vi "ReadSlotNode.vi"(8 "Error In":errorcluster, 11 "Slot Node In":refnum<k20>) -> (0 "Error Out":errorcluster, 2 "Slot Configuration":T1, 3 "Slot Node Out":refnum<k20>)   [LabVIEW 2012]
uses:
  SlotConfiguration.ctl
  BankConfiguration.ctl
  <vilib>/xml/NI_XML.lvlib
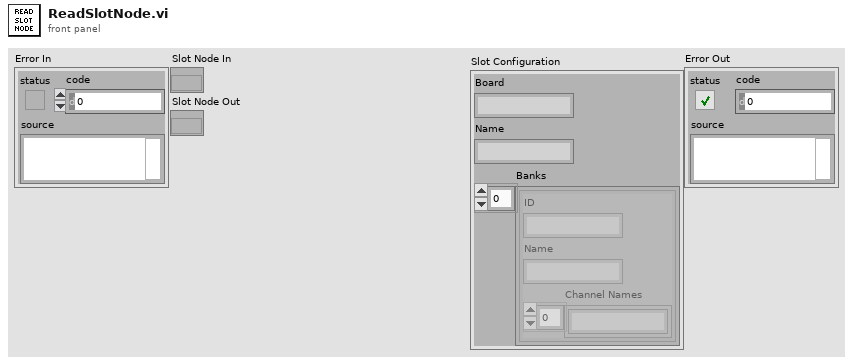
[diagram p1: front panel]
types:
  T1 = typedef "SlotConfiguration.ctl" = cluster{"Board":string, "Name":string, "Banks":T2[]}
  T2 = typedef "BankConfiguration.ctl" = cluster{"ID":string, "Name":string, "Channel Names":string[]}
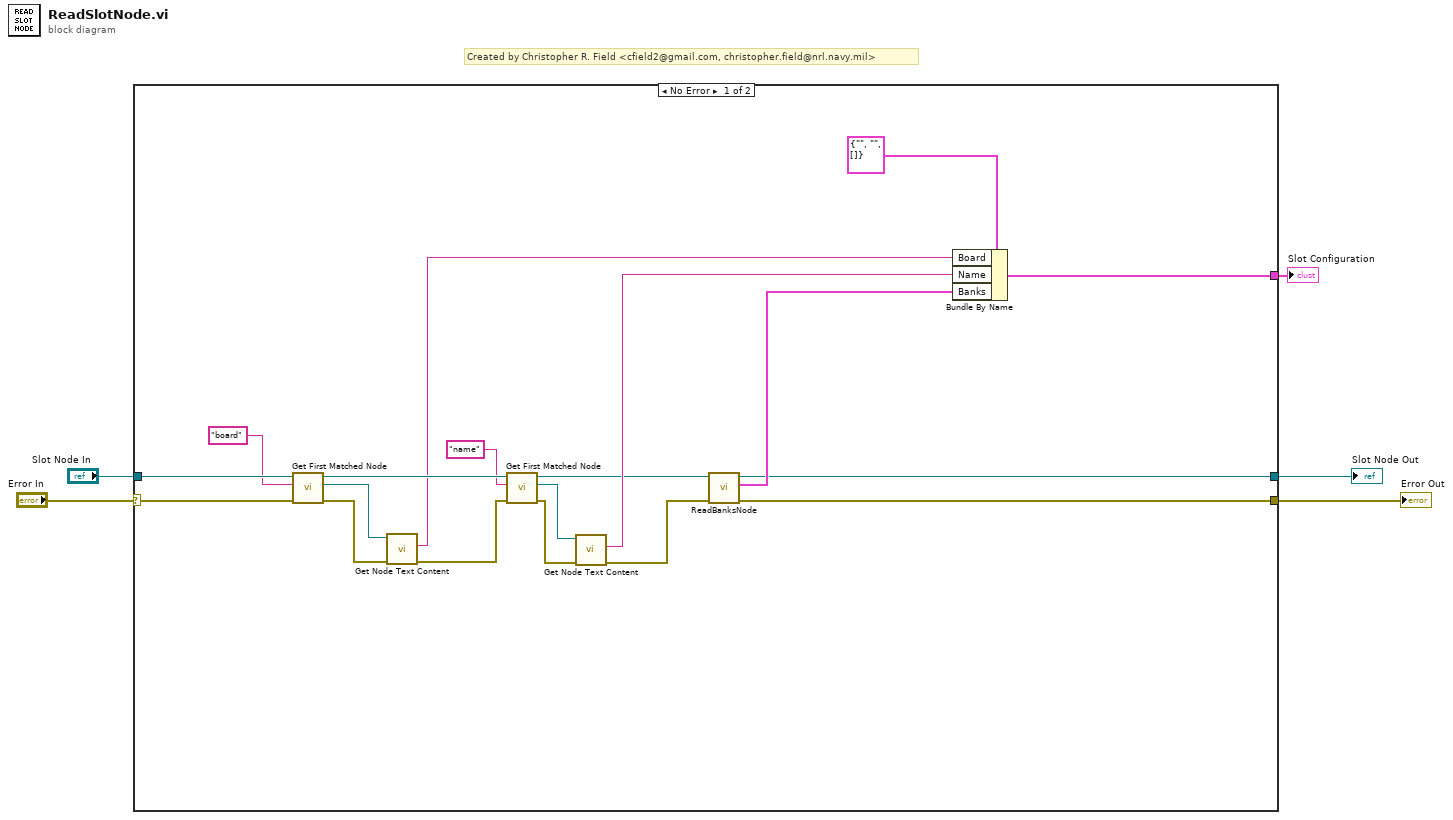
[diagram p0: block diagram]
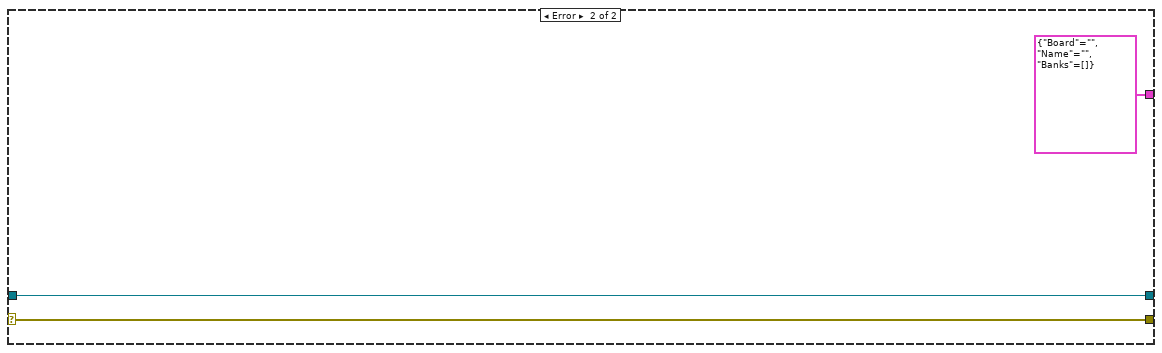
[diagram p2: hidden frame]
diagram:
  # "Created by Christopher R. Field <cfield2@gmail.com, christopher.field@nrl.navy.mil>"
  n1 = case shown="No Error" "Error In" {
    selector: "Error In" -> [w23 w26]
    tunnel: "Slot Node In" -> [w24 w27]
    tunnel: [w8 T1 {"Board"="", "Name"="", "Banks"=[]} ("Slot Configuration")] -> w3
    tunnel: [w7 w27] -> w1
    tunnel: [w6 w26] -> w2
    frame No Error {
      n2 = call <vilib>:"Get First Matched Node.vi"("error in (no error)"=w23, "XPath expression"="board", "node in"=w24) -> ("error out"=w20:errorcluster, "node result"=w21:refnum<k20>, "node out"=w19:refnum<k20>)  [unwired: 6 in]
      n3 = call <vilib>:"Get Node Text Content.vi"("error in (no error)"=w20, "node in"=w21) -> ("error out"=w17:errorcluster, "node text"=w13:string)  [unwired: 7 in, 1 out]
      n4 = call <vilib>:"Get First Matched Node.vi"("error in (no error)"=w17, "XPath expression"="name", "node in"=w19) -> ("error out"=w16:errorcluster, "node result"=w15:refnum<k20>, "node out"=w11:refnum<k20>)  [unwired: 6 in]
      n5 = call <vilib>:"Get Node Text Content.vi"("error in (no error)"=w16, "node in"=w15) -> ("error out"=w10:errorcluster, "node text"=w12:string)  [unwired: 7 in, 1 out]
      n6 = call "ReadBanksNode.vi"("Error In"=w10, "Slot Node In"=w11) -> ("Error Out"=w6:errorcluster, "Banks"=w9:T2[], "Slot Node Out"=w7:refnum<k20>)  [unwired: 7 in]
      n7 = Bundle By Name(cluster=T1 {"Board"="", "Name"="", "Banks"=[]} ("Slot Configuration"), "Board"=w13, "Name"=w12, "Banks"=w9) -> (w8:T1)
    }
    frame Error {
    }
  }
  "Slot Configuration" <- w3
  "Error Out" <- w2
  "Slot Node Out" <- w1
